vi "Close.vi"(0 "comm interface in":refnum<class "RoboRIO I2C.lvclass">, 11 "error in":errorcluster) -> (15 "error out":errorcluster)   [LabVIEW 2018, in "RoboRIO I2C.lvclass"]
uses:
  RoboRIO I2C.lvclass
  RoboRIO I2C.lvclass/RoboRIO I2C.ctl
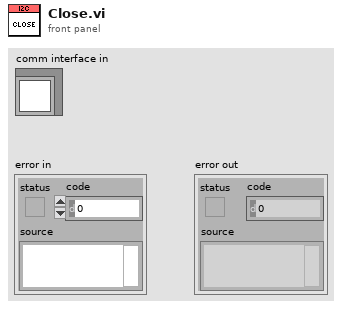
[diagram p1: front panel]
types:
  T1 = typedef "WPI_I2CDevRef.ctl" = cluster{"DevStatus":errorcluster, "Device Address":u8, "Handle":i32, "I2C Bus":T2}
  T2 = typedef "i2c_bus.ctl" = enum16{"I2C On-Board", "I2C MXP", "Invalid"}
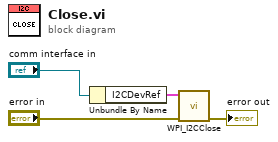
[diagram p0: block diagram]
diagram:
  n1 = Unbundle By Name("comm interface in") -> ("I2CDevRef"=w3:T1)
  n2 = call <vilib>:"WPI_I2CClose.vi"("error in (no error)"="error in", "I2CDevRef"=w3) -> ("error out"=→"error out":errorcluster)  [unwired: 9 in]
